vi "Choreo_Choreo_TrajectoryFromJSON.vi"(11 "JSON String":string) -> (0 "Error":bool, 3 "ChoreoTrajectory":T1)   [LabVIEW 2019]
doc: "Parse a choreo trajectory from a JSON formatted string. \n\nInputs: \n - JSON String - string- The string containing the choreo trajectory. Note that files may have a .TRAJ extension. These are actually internally formatted as JSON files.\n\nOutputs:\n - trajectory - cluster - Trajectory read from JSON file.\n - Error - boolean - TRUE if an error occured."
uses:
  TypeDef/ChoreoTrajectory.ctl
  TypeDef/ChoreoTrajectoryState.ctl
  ChoreoLib.lvlib
panel:
  in  "?":T3(array[cluster])
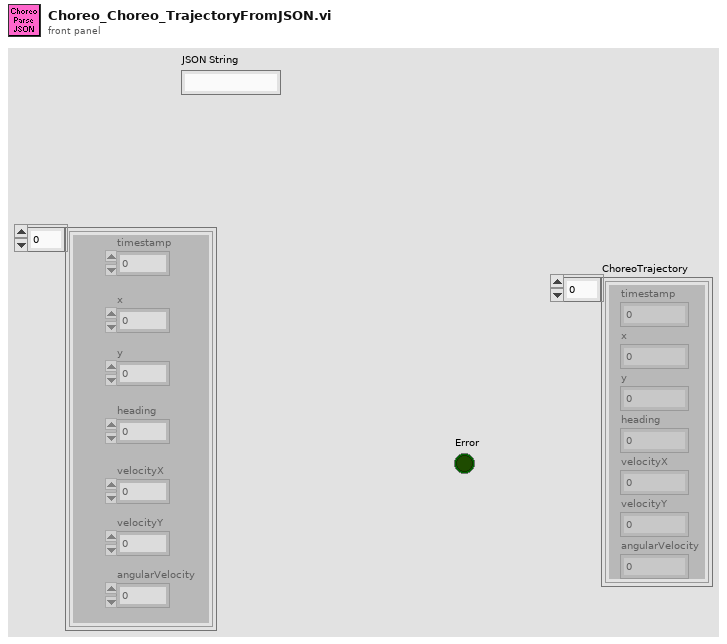
[diagram p1: front panel]
types:
  T1 = typedef "ChoreoLib.lvlib/ChoreoTrajectory.ctl" = T2[]
  T2 = typedef "ChoreoLib.lvlib/ChoreoTrajectoryState.ctl" = cluster{"timestamp":dbl, "x":dbl, "y":dbl, "heading":dbl, "velocityX":dbl, "velocityY":dbl, "angularVelocity":dbl}
  T3 = cluster{"timestamp":dbl, "x":dbl, "y":dbl, "heading":dbl, "velocityX":dbl, "velocityY":dbl, "angularVelocity":dbl}[]
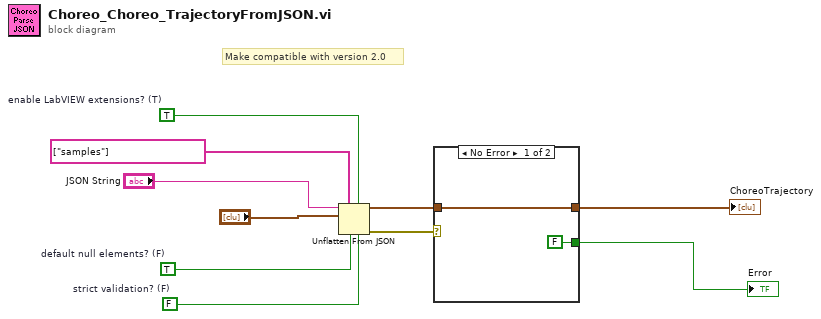
[diagram p0: block diagram]
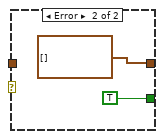
[diagram p2: hidden frame]
diagram:
  w5 = FALSE  # strict validation? (F)
  w6 = TRUE  # default null elements? (F)
  w8 = TRUE  # enable LabVIEW extensions? (T)
  # "Make compatible with version 2.0"
  n1 = Unflatten From JSON(path=string[] ["samples"] ("path 7"), enable LabVIEW extensions? (T)=w8, JSON string="JSON String", type and defaults="?", default null elements? (F)=w6, strict validation? (F)=w5) -> (value=w9:T3, error out=w10:errorcluster)  [unwired: 1 in]
  n2 = case shown="No Error" w10 {
    tunnel: w9 -> [w11 _]
    tunnel: [FALSE TRUE] -> w2
    tunnel: [w11 T1 [] ("ChoreoTrajectory 2")] -> w3
    frame No Error {
    }
    frame Error {
    }
  }
  "Error" <- w2
  "ChoreoTrajectory" <- w3
